vi "20170516-lecture4-2 prof OverrideButtonShortcutMenu.vi"() -> ()   [LabVIEW 2014]
doc: "This example shows how to display a context menu when you left-click a control. This example uses the Mouse Down? and Shortcut Menu Activation? filter events. In the Mouse Down? event, the example modifies the Button parameter so LabVIEW interprets a left-click as a right-click and fires the Shortcut Menu Activation? event."
panel:
  out "ItemTag":string
  in  "Stop":bool
  in  "Left-click or right-click on this control":u16
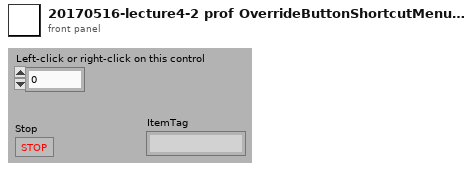
[diagram p1: front panel]
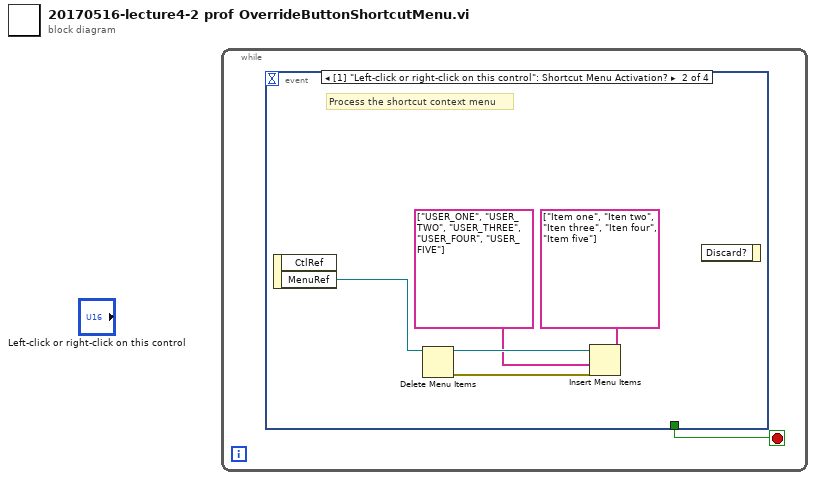
[diagram p0: block diagram]
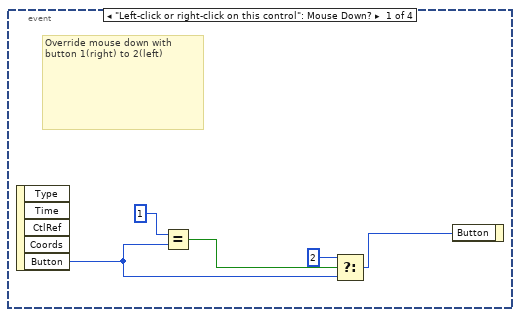
[diagram p2: hidden frame]
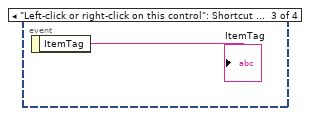
[diagram p3: hidden frame]
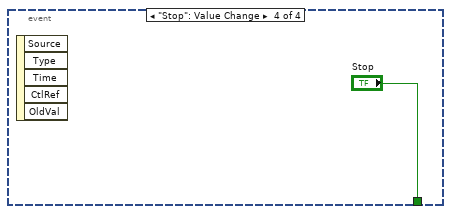
[diagram p4: hidden frame]
diagram:
  n1 = while {
    stop <- w1 stop-if-true
    n2 = event shown="[1] \"Left-click or right-click on this control\": Shortcut Menu Activation?" {
      selector: _ -> [_ _ _ _]
      dyn-events: _ -> [_ _ _ _]
      timeout: _ -> [_ _ _ _]
      tunnel: [_ _ _ "Stop"] -> w1
      event "Left-click or right-click on this control": Mouse Down? {
        # "Override mouse down with button 1(right) to 2(left)"
        n3 = event-data() -> ("Button"=w3:u16)  [unwired: 1 in, 4 out]
        n4 = Equal?(x=u16 1, y=w3) -> (x = y?=w2:bool)
        n5 = Select(t=u16 2, s=w2, f=w3) -> (s? t:f=w6:u16)
        n6 = event-data("Button"=w6) -> ()  [unwired: 1 in, 1 out]
      }
      event "Left-click or right-click on this control": Shortcut Menu Activation? {
        # "Process the shortcut context menu"
        n7 = event-data() -> ("MenuRef"=w11:refnum<k9>)  [unwired: 1 in, 1 out]
        n8 = Delete Menu Items(9:w11) -> (0:w8:errorcluster, 3:w10:refnum<k9>)  [unwired: 3 in]
        n9 = Insert Menu Items(6:w8, 7:string[] ["USER_ONE", "USER_TWO", "USER_THREE", "USER_FOUR", "USER_FIVE"], 8:string[] ["Item one", "Iten two", "Iten three", "Iten four", "Item five"], 9:w10) -> ()  [unwired: 2 in, 3 out]
        n10 = event-data() -> ()  [unwired: 2 in, 1 out]
      }
      event "Left-click or right-click on this control": Shortcut Menu Selection (User) {
        n11 = event-data() -> ("ItemTag"=→"ItemTag":string)  [unwired: 1 in]
      }
      event "Stop": Value Change {
        n12 = event-data() -> ()  [unwired: 1 in, 5 out]
      }
    }
  }
